vi "Plugin ID to Tree Items.vi"(8 "error in (no error)":errorcluster, 9 "Plugin ID":string, 11 "Application Data in":T2) -> (0 "error out":errorcluster, 1 "Settings":T1, 2 "Item":T1, 3 "Application Data out":T2)   [LabVIEW 2017, in "DSF Configuration Utility.lvlib"]
uses:
  DSF Configuration Utility.lvlib
  Main VI/Application Data.ctl
  VeriStand/Data Sharing Custom Device/Source/Engine/DSF Core.lvlibp/DSF Configuration API/Configuration Session.lvclass
  Main VI/View Mode.ctl
  Tree Item.ctl
  Tree Item Type.ctl
  VeriStand/Data Sharing Custom Device/Source/Engine/DSF Core.lvlibp/DSF Configuration API/Public/Read Item/Read Settings.vi
  VeriStand/Data Sharing Custom Device/Source/Engine/DSF Core.lvlibp/DSF Configuration API/Public/Read Item/Read Plugin.vi
panel:
  # "App\nData"
  # "App\nData"
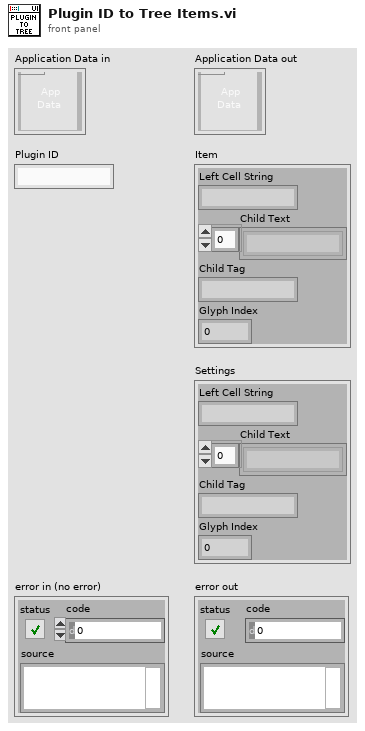
[diagram p1: front panel]
types:
  T1 = typedef "DSF Configuration Utility.lvlib/Tree Item.ctl" = cluster{"Left Cell String":string, "Child Text":string[], "Child Tag":string, "Glyph Index":i32}
  T2 = typedef "DSF Configuration Utility.lvlib/Application Data.ctl" = cluster{"Item Tree Control":refnum<vi>, "Value Tree Control":refnum<vi>, "DSF Refnum":refnum<class "Configuration Session.lvclass">, "Top-Level VI":refnum<vi>, "View State":T3, "menu reference":refnum<k9>}
  T3 = typedef "DSF Configuration Utility.lvlib/View Mode.ctl" = enum16{"Tree", "List"}
  T4 = typedef "DSF Configuration Utility.lvlib/Tree Item Type.ctl" = enum16{"Plugin", "Group", "Transfer", "Channel", "Setting"}
  T5 = typedef "DSF Core.lvlibp/DSF Plugin Info.ctl" = cluster{"components":string[], "timing":T6, "group ids":string[], "settings id":string, "threads":T7[]}
  T6 = typedef "DSF Core.lvlibp/DSF Timing Info.ctl" = cluster{"priority":u64, "decimation":u64, "offset":u64}
  T7 = typedef "DSF Core.lvlibp/DSF Engine Plugin Thread Configuration.ctl" = cluster{"buffer converter settings":T8, "transceiver settings":T8, "processor":i32, "priority offset":i16}
  T8 = typedef "DSF Core.lvlibp/DSF Settings Info.ctl" = cluster{"key":string, "value":string}[]
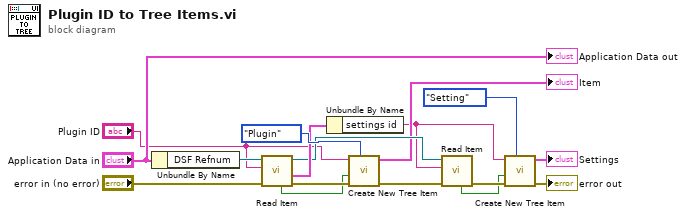
[diagram p0: block diagram]
diagram:
  n1 = Unbundle By Name("Application Data in") -> ("DSF Refnum"=w9:refnum<class "Configuration Session.lvclass">)
  n2 = call-poly "Read Item.vi"("error in (no error)"="error in (no error)", "Plugin ID"="Plugin ID", "Configuration Session in"=w9) -> ("error out"=w12:errorcluster, "value"=w14:T5, "Configuration Session out"=w8:refnum<class "Configuration Session.lvclass">, "found?"=w3:bool)  [unwired: 5 in]
  n3 = Unbundle By Name(w14) -> ("settings id"=w1:string)
  n4 = call "Create New Tree Item.vi"("Item Type"=Tree_Item_Type."Plugin", "error in"=w12, "found?"=w3, "Left Cell String"="Plugin ID") -> ("error out"=w11:errorcluster, "Item"=→"Item":T1)  [unwired: 6 in]
  n5 = call-poly "Read Item.vi"("error in (no error)"=w11, "Settings ID"=w1, "Configuration Session in"=w8) -> ("error out"=w15:errorcluster, "found?"=w4:bool)  [unwired: 5 in, 2 out]
  n6 = call "Create New Tree Item.vi"("Item Type"=Tree_Item_Type."Setting", "error in"=w15, "found?"=w4, "Left Cell String"=w1) -> ("error out"=→"error out":errorcluster, "Item"=→"Settings":T1)  [unwired: 6 in]
  "Application Data out" <- "Application Data in"
